vi "StromBrennweite.vi"(8 "f_max":dbl=200.0, 9 "f_min":dbl=80.0, 10 "f_offset":dbl=99999.0, 11 "f_var":dbl=200.0) -> (1 "I_var_1":dbl=294.1354035926154, 2 "D1":dbl, 3 "f_ges":dbl)   [LabVIEW 2013]
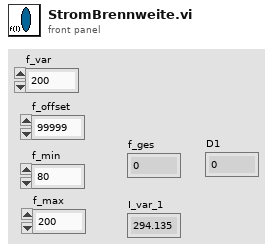
[diagram p1: front panel]
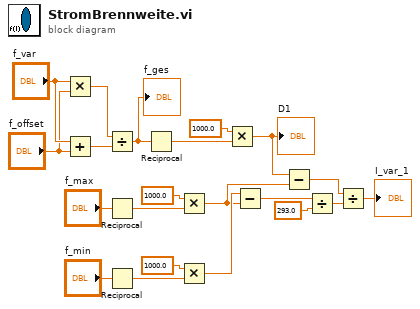
[diagram p0: block diagram]
diagram:
  n1 = Multiply(x="f_var", y="f_offset") -> (x*y=w20:dbl)
  n2 = Add(x="f_var", y="f_offset") -> (x+y=w21:dbl)
  n3 = Divide(x=w20, y=w21) -> (x/y=w5:dbl)
  "f_ges" <- w5
  n4 = Reciprocal(x="f_max") -> (1/x=w14:dbl)
  n5 = Reciprocal(x="f_min") -> (1/x=w16:dbl)
  n6 = Reciprocal(x=w5) -> (1/x=w18:dbl)
  n7 = Multiply(x=1000.0, y=w14) -> (x*y=w4:dbl)
  n8 = Multiply(x=1000.0, y=w16) -> (x*y=w12:dbl)
  n9 = Multiply(x=1000.0, y=w18) -> (x*y=w11:dbl)
  "D1" <- w11
  n10 = Subtract(x=w12, y=w4) -> (x-y=w7:dbl)
  n11 = Subtract(x=w11, y=w4) -> (x-y=w10:dbl)
  n12 = Divide(x=w7, y=293.0 ("x")) -> (x/y=w8:dbl)
  n13 = Divide(x=w10, y=w8) -> (x/y=→"I_var_1":dbl)
